vi "rad_Verify Image Compatibility.vi"(6 "Require Identical Chassis?":bool, 7 "Password":string, 8 "error in (no error)":errorcluster, 10 "Target address":T4={"Hostname"="", "Serial number"="", "Product name"="", "Product code"=0, "System status"="", "Credential type"=enum."None/Unlocked", "User added?"=FALSE, "Primary NIC"={"MAC address"="", "IP Address Request Mode"=2, "IP address"="", "Subnet mask"="", "Gateway"="", "DNS server"=""}} {"Primary NIC"."IP Address Request Mode" items=["Static"=1, "DHCP/Link-Local"=2, "Link-Local Only"=4, "DHCP Only"=8]}, 11 "AppImage Properties":T1) -> (0 "error out":errorcluster, 3 "Compatible?":bool, 5 "Status message":string)   [LabVIEW 2020]
uses:
  TypeDefs/rad_Application Image Properties.ctl
  TypeDefs/rad_FPGA Properties.ctl
  TypeDefs/rad_FPGA Flash Properties.ctl
  Targets/TypeDefs/rad_Target Network Settings.ctl
  Targets/TypeDefs/rad_Target Information.ctl
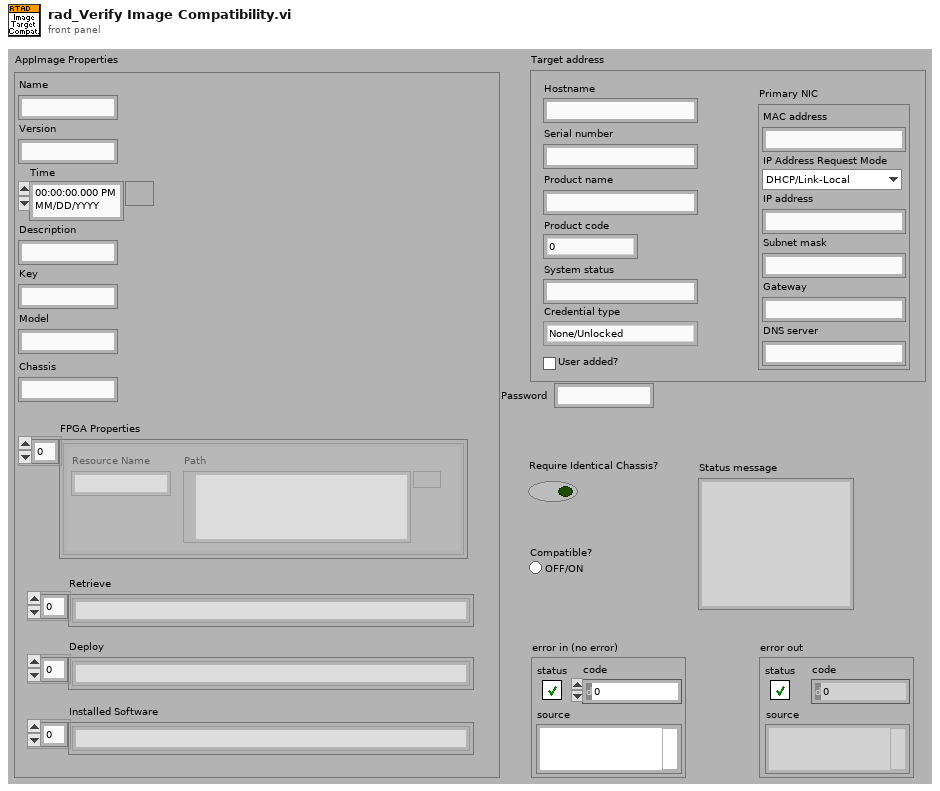
[diagram p1: front panel]
types:
  T1 = typedef "rad_Application Image Properties.ctl" = cluster{"Name":string, "Version":string, "Time":timestamp, "Description":string, "Key":string, "Chassis":string, "FPGA Properties":T2, "Model":string, "Retrieve":string[], "Deploy":string[], "Installed Software":string[]}
  T2 = typedef "rad_FPGA Properties.ctl" = T3[]
  T3 = typedef "rad_FPGA Flash Properties.ctl" = cluster{"Resource Name":string, "Path":path}
  T4 = typedef "rad_Target Information.ctl" = cluster{"Hostname":string, "Serial number":string, "Product name":string, "Product code":i32, "System status":string, "Credential type":enum16{"None/Unlocked", "FTP Password", "NIAuth Credentials"}, "User added?":bool, "Primary NIC":T5}
  T5 = typedef "rad_Target Network Settings.ctl" = cluster{"MAC address":string, "IP Address Request Mode":i32, "IP address":string, "Subnet mask":string, "Gateway":string, "DNS server":string}
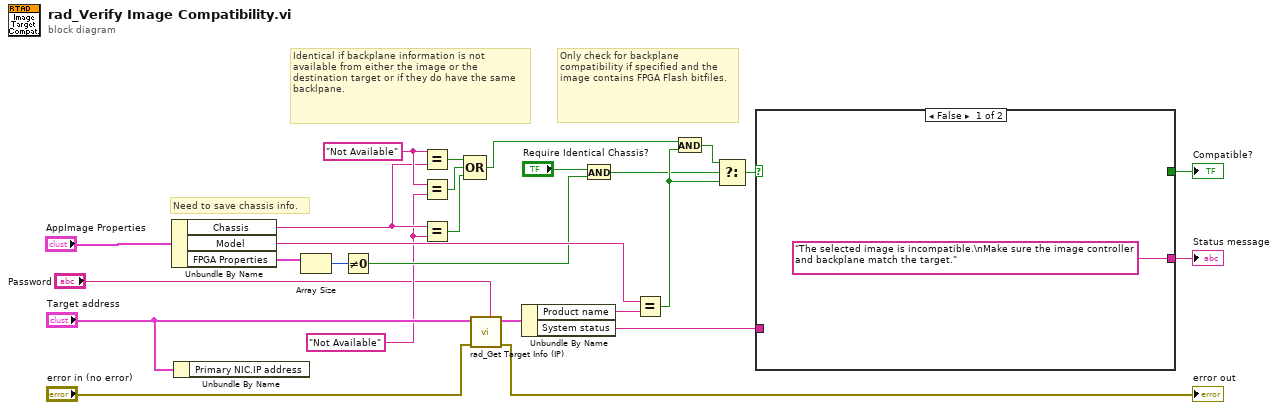
[diagram p0: block diagram]
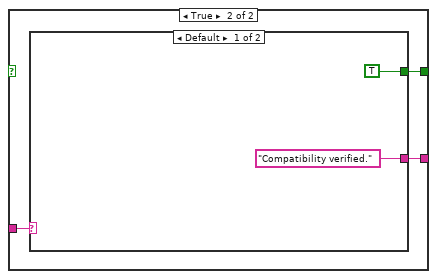
[diagram p2: hidden frame]
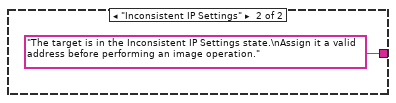
[diagram p3: hidden frame]
diagram:
  w3 = "Not Available"
  w22 = "Not Available"
  # "Only check for backplane compatibility if specified and the image contains FPGA Flash bitfiles."
  # "Identical if backplane information is not available from either the image or the destination target or if they do have the same backlpane."
  # "Need to save chassis info."
  n1 = Unbundle By Name("AppImage Properties") -> ("Chassis"=w21:string, "Model"=w23:string, "FPGA Properties"=w14:T2)
  n2 = Unbundle By Name("Target address") -> ()  [unwired: 1 out]
  n3 = Array Size(array=w14) -> (size(s)=w13:i32)
  n4 = Not Equal To 0?(x=w13) -> (x != 0?=w11:bool)
  n5 = Equal?(x=w22, y=w21) -> (x = y?=w20:bool)
  n6 = Equal?(x=w22, y=w3) -> (x = y?=w19:bool)
  n7 = Equal?(x=w21, y=w3) -> (x = y?=w18:bool)
  n8 = Compound Arithmetic op=OR(w20, w19, w18) -> (w17:bool)
  n9 = call "rad_Get Target Info (IP).vi"("Password"="Password", "error in (no error)"="error in (no error)", "Target settings in"="Target address") -> ("error out"=→"error out":errorcluster, "Target settings out"=w15:T4)  [unwired: 7 in]
  n10 = Unbundle By Name(w15) -> ("Product name"=w26:string, "System status"=w5:string)
  n11 = And(x="Require Identical Chassis?", y=w11) -> (x .and. y?=w10:bool)
  n12 = Equal?(x=w23, y=w26) -> (x = y?=w25:bool)
  n13 = And(x=w17, y=w25) -> (x .and. y?=w24:bool)
  n14 = Select(t=w24, s=w10, f=w25) -> (s? t:f=w8:bool)
  n15 = case shown="False" w8 {
    tunnel: [_ w29] -> w7
    tunnel: ["The selected image is incompatible.\nMake sure the image controller and backplane match the target." w28] -> w6
    tunnel: w5 -> [_ w30]
    frame False {
    }
    frame True {
      n16 = case shown="Default" w30 {
        tunnel: [TRUE _] -> w29
        tunnel: ["Compatibility verified." ("f") "The target is in the Inconsistent IP Settings state.\nAssign it a valid address before performing an image operation."] -> w28
        frame Default {
        }
        frame "Inconsistent IP Settings" {
        }
      }
    }
  }
  "Compatible?" <- w7
  "Status message" <- w6
